vi "MCL Change Clock.vi"(9 "handle":i32, 10 "clock":i16, 11 "milliseconds":dbl) -> (3 "function return":i32)   [LabVIEW 2017, in "Madlib.lvlib"]
doc: "MADLIB_API int MCL_ChangeClock(double milliseconds, short clock, int handle);"
uses:
  Madlib.lvlib
  Madlib.dll
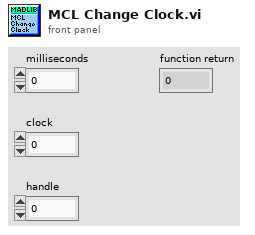
[diagram p1: front panel]
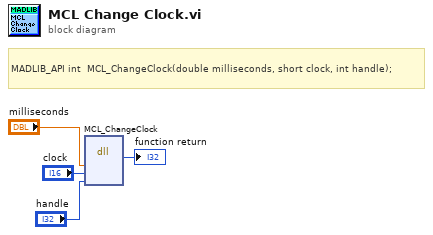
[diagram p0: block diagram]
diagram:
  # "MADLIB_API\tint\t\tMCL_ChangeClock(double milliseconds, short clock, int handle);"
  n1 = dll-call lib="C:/Users/francesco/dev/pump-probe/Piezo/lvlib/Madlib.*" fn="MCL_ChangeClock"("milliseconds"="milliseconds", "clock"="clock", "handle"="handle") -> (→"function return":i32)  [unwired: 6 in, 2 out]
